vi "Get - Fs.vi"(0 "reference in":refnum<class "GSwFormDSP.lvclass">, 5 "error in (no error)":errorcluster) -> (11 "Nb Different Fs":i32, 13 "Signals Fs":dbl[](array[numeric]), 14 "reference in":refnum<class "GSwFormDSP.lvclass">, 19 "error out":errorcluster)   [LabVIEW 2022 SP3, in "GSwFormDSP.lvclass"]
uses:
  GSwFormDSP.lvclass
  Generic Utilities_class/Generic Utilities.lvclass
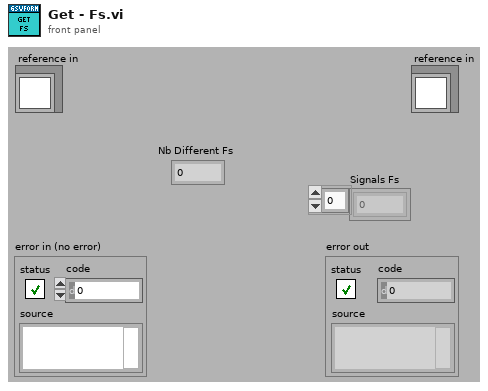
[diagram p1: front panel]
types:
  T1 = typedef "GSwFormDSP.lvclass/ObjectAttributes.ctl" = cluster{"Wform Ref":refnum<data-value>, "Nb Signals":i32, "Spectral Function Parameters":T2, "FFT":waveform(cdb)[], "Nb FFT":i32, "Nb Averages":i32[], "Reference Indexes":i32[], "Response Indexes":i32[], "Coherence":waveform(dbl)[], "TDF Parameters":T4, "DAQ":cluster{"Duration (sec)":dbl, "Buffer Size (Samples)":i32, "Offset (Samples)":i32}, "Filter Impulse Response (TDF)":waveform(dbl), "Sound Playback":T5}
  T2 = typedef "GSwFormDSP.lvclass/Spectral Parameters.ctl" = cluster{"Frequency resolution (Hz)":dbl, "Overlap":dbl, "Window":T3}
  T3 = typedef "NI_AALPro.lvlib/windowTd.ctl" = u32
  T4 = typedef "GSwFormDSP.lvclass/TDF Parameters.ctl" = cluster{"Filter":enum32{"Lowpass", "Highpass", "Bandpass", "Bandstop"}, "Type:":enum16{"Butterworth", "Chebyshev", "Inv Chebyshev", "Elliptic", "Bessel"}, "LP cutoff freq":dbl, "HP cutoff freq":dbl, "Order":i32, "passband ripple (dB)":dbl, "stopband attenuation (dB)":dbl, "Phaseless Filter":bool, "Include Fade IN and OUT":bool}
  T5 = typedef "GSwFormDSP.lvclass/Sound Playback.ctl" = cluster{"Timer start (ms)":u32, "task ID":T6, "Cursor Init Location (s)":dbl, "SC Volume":dbl}
  T6 = typedef "Sound Output Task ID.ctl" = u32
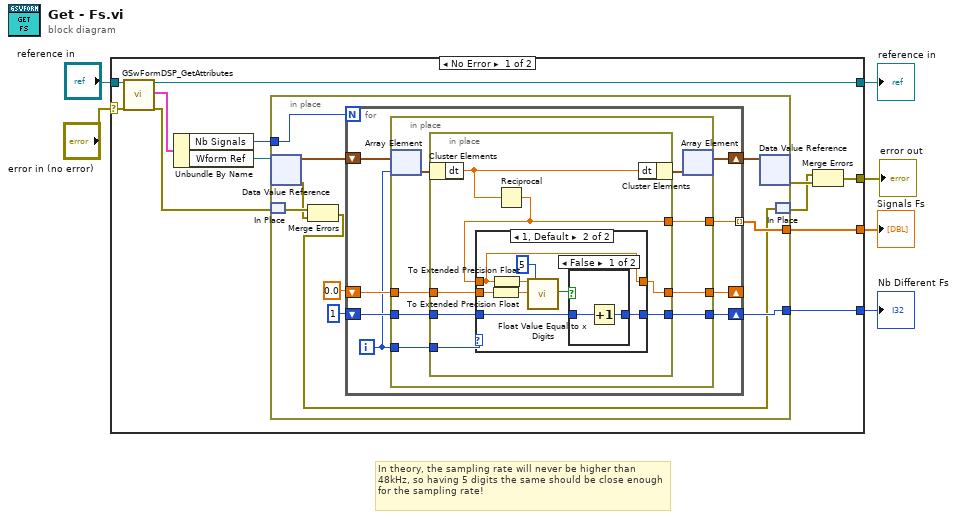
[diagram p0: block diagram]
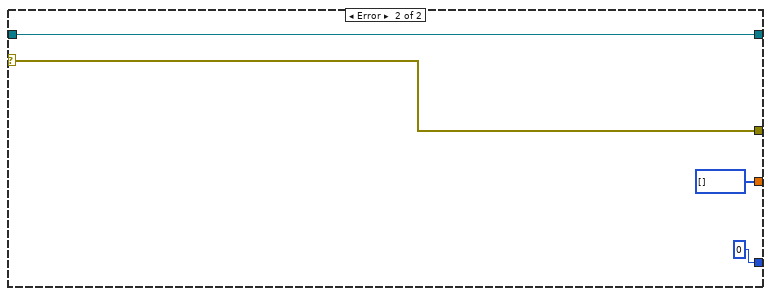
[diagram p4: hidden frame]
diagram:
  # "In theory, the sampling rate will never be higher than 48kHz, so having 5 digits the same should be close enough for the sampling rate!"
  n1 = case shown="No Error" "error in (no error)" {
    selector: "error in (no error)" -> [w13 w68]
    tunnel: [w16 w68] -> w5
    tunnel: [w14 w67] -> w3
    tunnel: "reference in" -> [w15 w67]
    tunnel: [w18 i32[] []] -> w2
    tunnel: [w17 0] -> w1
    frame No Error {
      n2 = call "GSwFormDSP_GetAttributes.vi"("reference in"=w15, "error in (no error)"=w13) -> ("reference out"=w14:refnum<class "GSwFormDSP.lvclass">, "attributes"=w12:T1, "error out"=w10:errorcluster)  [unwired: 14 in, 1 out]
      n3 = Unbundle By Name(w12) -> ("Nb Signals"=w9:i32, "Wform Ref"=w11:refnum<data-value>)
      n4 = in-place {
        in-place-border: [w27] -> w18
        in-place-border: [w24] -> w17
        in-place-border: w9 -> [w20]
        n5 = in-place-dvr #1(w11) -> (w28:waveform(dbl)[], w21:errorcluster)
        n6 = in-place-match #2(w10) -> (w22:errorcluster)
        n7 = Merge Errors(w22, w21) -> (w19:errorcluster)
        n8 = for {
          N: w20 -> [_]
          tunnel: [w32] -> w27 mode=indexing
          shift-right: [w36] -> _
          shift-left: 0.0 ("Fs") -> [w35]
          shift-right: [w34] -> w24
          shift-left: 1 -> [w33]
          shift-right: [w29] -> w23
          shift-left: w28 -> [w31]
          i -> [w30]
          n9 = in-place {
            in-place-border: w30 -> [w44]
            in-place-border: [w43] -> w36
            in-place-border: w35 -> [w42]
            in-place-border: [w41] -> w34
            in-place-border: w33 -> [w40]
            in-place-border: [w39] -> w32
            n10 = in-place-array #3(w31, w30) -> (w38:waveform(dbl))
            n11 = in-place {
              in-place-border: w44 -> [w51]
              in-place-border: [w50] -> w43
              in-place-border: w42 -> [w49]
              in-place-border: [w48] -> w41
              in-place-border: w40 -> [w47]
              in-place-border: [w45] -> w39
              n12 = in-place-cluster #4(w38) -> ("dt"=w46:dbl)
              n13 = Reciprocal(x=w46) -> (1/x=w45:dbl)
              n14 = case shown="1, Default" w51 {
                tunnel: [w53 w59] -> w50
                tunnel: w45 -> [w53 w59]
                tunnel: w49 -> [_ w58]
                tunnel: [w52 w61] -> w48
                tunnel: w47 -> [w52 w60]
                frame 0 {
                }
                frame 1, Default {
                  n15 = To Extended Precision Float(1:w58) -> (0:w55:ext)
                  n16 = To Extended Precision Float(1:w59) -> (0:w56:ext)
                  n17 = call "Float Value Equal to x Digits.vi"("Value A"=w56, "Value B"=w55, "Desired Number of matching digits"=5) -> ("Equal?"=w57:bool)  [unwired: 16 in]
                  n18 = case shown="False" w57 {
                    tunnel: [w63 w64] -> w61
                    tunnel: w60 -> [w62 w64]
                    frame False {
                      n19 = Increment(x=w62) -> (x+1=w63:i32)
                    }
                    frame True {
                    }
                  }
                }
              }
              n20 = in-place-cluster #4("dt"=w46) -> (w37:waveform(dbl))
            }
            n21 = in-place-array #3(w37) -> (w29:waveform(dbl)[])  [unwired: 1 out]
          }
        }
        n22 = in-place-dvr #1(w23) -> (w8:errorcluster)  [unwired: 1 out]
        n23 = in-place-match #2(w19) -> (w7:errorcluster)
      }
      n24 = Merge Errors(w7, w8) -> (w16:errorcluster)
    }
    frame Error {
    }
  }
  "error out" <- w5
  "reference in" <- w3
  "Signals Fs" <- w2
  "Nb Different Fs" <- w1
